vi "Example Cluster 1.vi"() -> ()   [LabVIEW 2014]
uses:
  utils 2/PointerDatatype.lvclass
  utils 2/PointerInt32Datatype.lvclass
  utils 2/PointerStringDatatype.lvclass
  ClusterTypedef1.ctl
panel:
  out "output cluster":T1
  out "Error Out":errorcluster
  in  "Error In":errorcluster
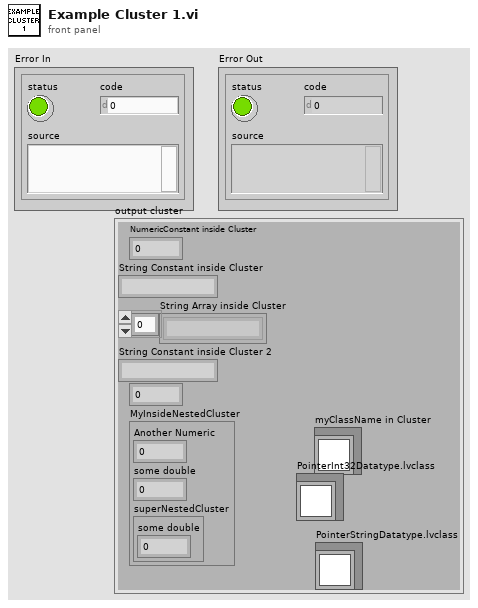
[diagram p1: front panel]
types:
  T1 = cluster{"NumericConstant inside Cluster":i32, "String Constant inside Cluster":string, "String Array inside Cluster":string[], "String Constant inside Cluster 2":string, dbl, "MyInsideNestedCluster":cluster{"Another Numeric":i32, "some double":dbl, "superNestedCluster":cluster{"some double":dbl}}, "myClassName in Cluster":refnum<class "PointerDatatype.lvclass">, "PointerInt32Datatype.lvclass":refnum<class "PointerInt32Datatype.lvclass">, "PointerStringDatatype.lvclass":refnum<class "PointerStringDatatype.lvclass">}
  T2 = typedef "ClusterTypedef1.ctl" = cluster{"some double":dbl}
  T3 = cluster{"NumericConstant inside Cluster":i32, "String Constant inside Cluster":string, "String Array inside Cluster":string[], "String Constant inside Cluster 2":string, dbl, "MyInsideNestedCluster":cluster{"Another Numeric":i32, "some double":dbl, "superNestedCluster":T2}, "myClassName in Cluster":refnum<class "PointerDatatype.lvclass">, "PointerInt32Datatype.lvclass":refnum<class "PointerInt32Datatype.lvclass">, "PointerStringDatatype.lvclass":refnum<class "PointerStringDatatype.lvclass">}
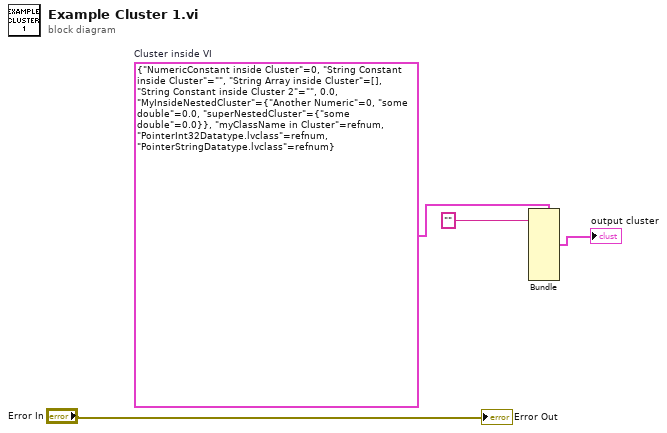
[diagram p0: block diagram]
diagram:
  w3 = T3 {"NumericConstant inside Cluster"=0, "String Constant inside Cluster"="", "String Array inside Cluster"=[], "String Constant inside Cluster 2"="", 0.0, "MyInsideNestedCluster"={"Another Numeric"=0, "some double"=0.0, "superNestedCluster"={"some double"=0.0}}, "myClassName in Cluster"=refnum, "PointerInt32Datatype.lvclass"=refnum, "PointerStringDatatype.lvclass"=refnum}  # Cluster inside VI
  n1 = Bundle(cluster=w3, "String Constant inside Cluster"="") -> (→"output cluster":T3)  [unwired: 8 in]
  "Error Out" <- "Error In"
